vi "PECT - Scan_time gate_counter - PCI6071E.vi"() -> ()   [LabVIEW 2012]
uses:
  <vilib>/DAQmx/read.llb/DAQmx Read (Digital Bool 1Line 1Point).vi
  <vilib>/DAQmx/read.llb/DAQmx Read (Analog 2D DBL NChan NSamp).vi
  <vilib>/Instr/_visa.llb/VISA Configure Serial Port (Instr).vi
  <vilib>/DAQmx/create/channels.llb/DAQmx Create Channel (CO-Pulse Generation-Frequency).vi
  <vilib>/DAQmx/configure/timing.llb/DAQmx Timing (Implicit).vi
  <vilib>/DAQmx/configure/trigger.llb/DAQmx Start Trigger (Digital Edge).vi
  <vilib>/DAQmx/create/channels.llb/DAQmx Create Channel (DI-Digital Input).vi
  <vilib>/DAQmx/create/channels.llb/DAQmx Create Channel (AI-Voltage-Basic).vi
  <vilib>/DAQmx/configure/timing.llb/DAQmx Timing (Sample Clock).vi
  <vilib>/DAQmx/miscellaneous.llb/DAQmx Fill In Error Info.vi
  <resource>/objmgr/daqmx.rc
  <vilib>/Platform/NI_3dgraph.lvlib
  <vilib>/DAQmx/read.llb/DAQmx Read (Counter U32 1Chan 1Samp).vi
  <vilib>/DAQmx/create/channels.llb/DAQmx Create Channel (CI-Count Edges).vi
panel:
  in  "Counter Terminal":tag="/Dev3/PFI3"
  in  "Counter source":tag="Dev3/ctr1"
  in  "Tab Control 3":enum32{"Control", "Data Processing"}(tab)
  in  "Backdata online":bool caption="Scan"
  in  "Offset":bool
  in  "Open csv":bool
  in  "Scan":bool
  in  "Save Scan mode":bool caption="Save Process"
  in  "Gate 1":dbl=3.0
  in  "Gate 2":dbl=25.0
  in  "Stop Scan":bool
  in  "Right":bool
  in  "Left":bool
  in  "Front":bool
  in  "Back":bool
  in  "Home X":bool
  in  "Home Y":bool
  in  "Stop 3":bool
  in  "Emergency Stop":bool
  in  "Move Distance":dbl=5.0
  in  "Open tdms":bool
  in  "Pulse frequency":dbl=1000.0 format="%0.2p"
  in  "Pulser Cycles":i32=10
  in  "Sensor No.":i32
  in  "Graph":bool
  in  "Sensor Index":dbl[](array[numeric])=[5.0, 10.0, 12.0, 15.0, 19.0]
  in  "Inverse":bool caption="Scan"
  in  "Trim data":bool caption="Scan"
  in  "X-min":dbl
  in  "X-max":dbl
  in  "Y-min":dbl
  in  "Y-max":dbl
  in  "ViewMode":i32(ring) items=["cwViewXYPlane", "cwViewXZPlane", "cwViewYZPlane", "cwViewUserDefined"]
  in  "Plot style":i32(ring)=5 items=["cwLine"=1, "cwPoint"=2, "cwLinePoint"=3, "cwHiddenLine"=4, "cwSurface"=5, "cwSurfaceLine"=6, "cwSurfaceNormal"=7, "cwContourLine"=8, "cwSurfaceContour"=9]
  in  "Repair Line Col":bool
  in  "Repair Line Row":bool
  in  "Line Col":dbl=167.0
  in  "Line Row":dbl
  in  "low cutoff freq":dbl=40.0 format="%0.2f"
  in  "Filter":bool caption="Scan"
  in  "Backdata":bool caption="Scan"
  in  "Odd":bool caption="Scan"
  in  "DiffY":bool caption="Scan"
  in  "DiffX":bool caption="Scan"
  in  "ColorMapAutoScale":bool=TRUE
  in  "Max":dbl=0.6
  in  "Min":dbl=-0.8
  in  "Abs":bool caption="Scan"
  in  "Backindex":i32
  out "Completed":bool
  out "Start Pos. X":dbl=-55.0 format="%#.4f"
  out "Start. Pos.Y":dbl=-76.83 format="%#.4f"
  in  "Tab Control 2":T1(tab)
  out "Hall sensors signal":dbl[][](graph)
  out "Feature Extraction":dbl(graph)
  in  "3D Surface":refnum<k7>(container)
  out "Record path":path caption="selected path"
  out "Feature extraction scan":dbl[](graph)
  in  "Tab Control":T2(tab)=enum."          DAQ        "
  in  "Step X":dbl=0.5
  out "Move X":bool
  in  "Direction (+)":bool=TRUE
  in  "Step Y":dbl=1.0
  in  "Y-length":dbl=1.0
  in  "X-length":dbl=30.0
  in  "Save Speed":bool
  in  "Cur. Pos Y":dbl=18.8 format="%#.4f"
  in  "Cur. Pos X":dbl=-22.5 format="%#.4f"
  in  "Travel per Pulse (mm)":dbl=0.002
  in  "2 Rate":dbl=0.2
  in  "1 Rate":dbl=0.2
  in  "2 Min":dbl=1.0
  in  "1  Max":dbl=8.0
  in  "2 Max":dbl=8.0
  in  "1 Min":dbl=1.0
  in  "Parity":u16(ring) items=["None", "Odd", "Even", "Mark", "Space"]
  in  "stop bits":u16(ring)=10 items=["1.0"=10, "1.5"=15, "2.0"=20]
  in  "Data bits":u16=8 min=5 max=8 step=1
  in  "Baud Rate":u32=9600
  in  "COM Port":refnum<visa-resource-name>="COM3"
  out "No. X":i32
  out "No. Y":i32
  out "No. Data":i32
  out "Counter Status":bool
  out "Motor Pulse Count":i32
  in  "Digital Sampling Rate":dbl=1000.0
  in  "Digital Line":tag="Dev3/port0/line0"
  in  "AI Sample Clock":tag="/Dev3/Ctr0InternalOutput"
  in  "Pulse Counter":tag="Dev3/ctr0"
  in  "Edge":i32(ring)=10280 items=["Rising"=10280, "Falling"=10171]
  in  "Pulser edge terminal":tag="/Dev3/PFI0"
  out "Sample per Channel AI":dbl
  out "Actual Sample Rate":dbl=500000.0 format="%0.2f"
  in  "Physical Channel":tag="Dev3/ai0:31"
  in  "Min Voltage":dbl=-10.0
  in  "Max Voltage":dbl=10.0
  in  "Terminal Configuration":i32(ring)=10083 items=["default"=-1, "RSE"=10083, "NRSE"=10078, "Differential"=10106, "Pseudodifferential"=12529]
  in  "Sample Rate":dbl=30000.0
  in  "Save Scan mode 2":bool caption="Save Process"
  # "Pulse setting"
  # "Data Processing"
  # "Time gate = %T/2"
  # "Motor control"
  # "Color map"
  # "Process"
  # "Repair line"
  # "Hall Sensors Signal"
  # "Feature Extraction"
  # "COM  Setting"
  # "Speed  Setting"
  # "Scan  Setting"
  # "Pulser"
  # "Motor Trigger"
  # "Sensor  Channel"
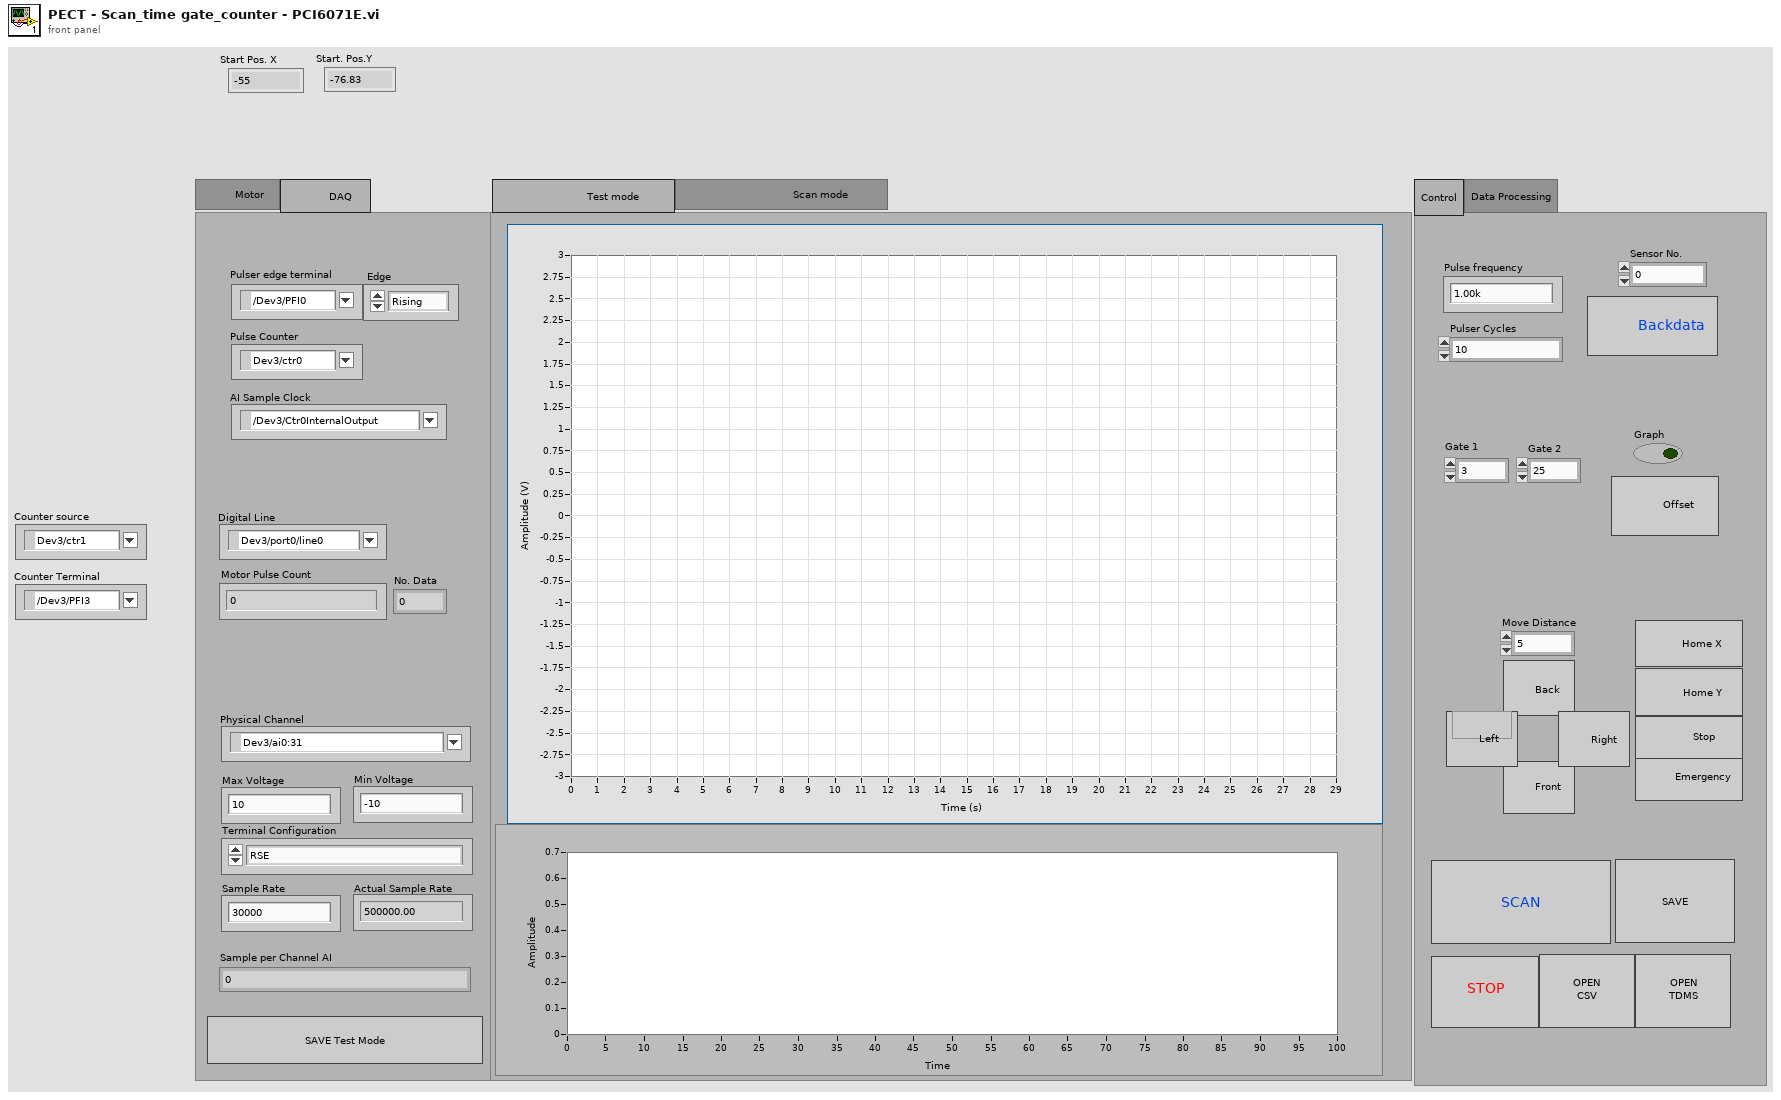
[diagram p1: front panel]
types:
  T1 = enum32{"                    Test mode                   ", "                          Scan mode                      "}
  T2 = enum32{"        Motor      ", "          DAQ        "}
  T3 = enum16{"No Scan", "Move X", "Wait to destination X", "Move Y", "Wait to destinatioin Y"}
  T4 = enum16{"open", "open or create", "create or replace", "create", "open (read-only)"}
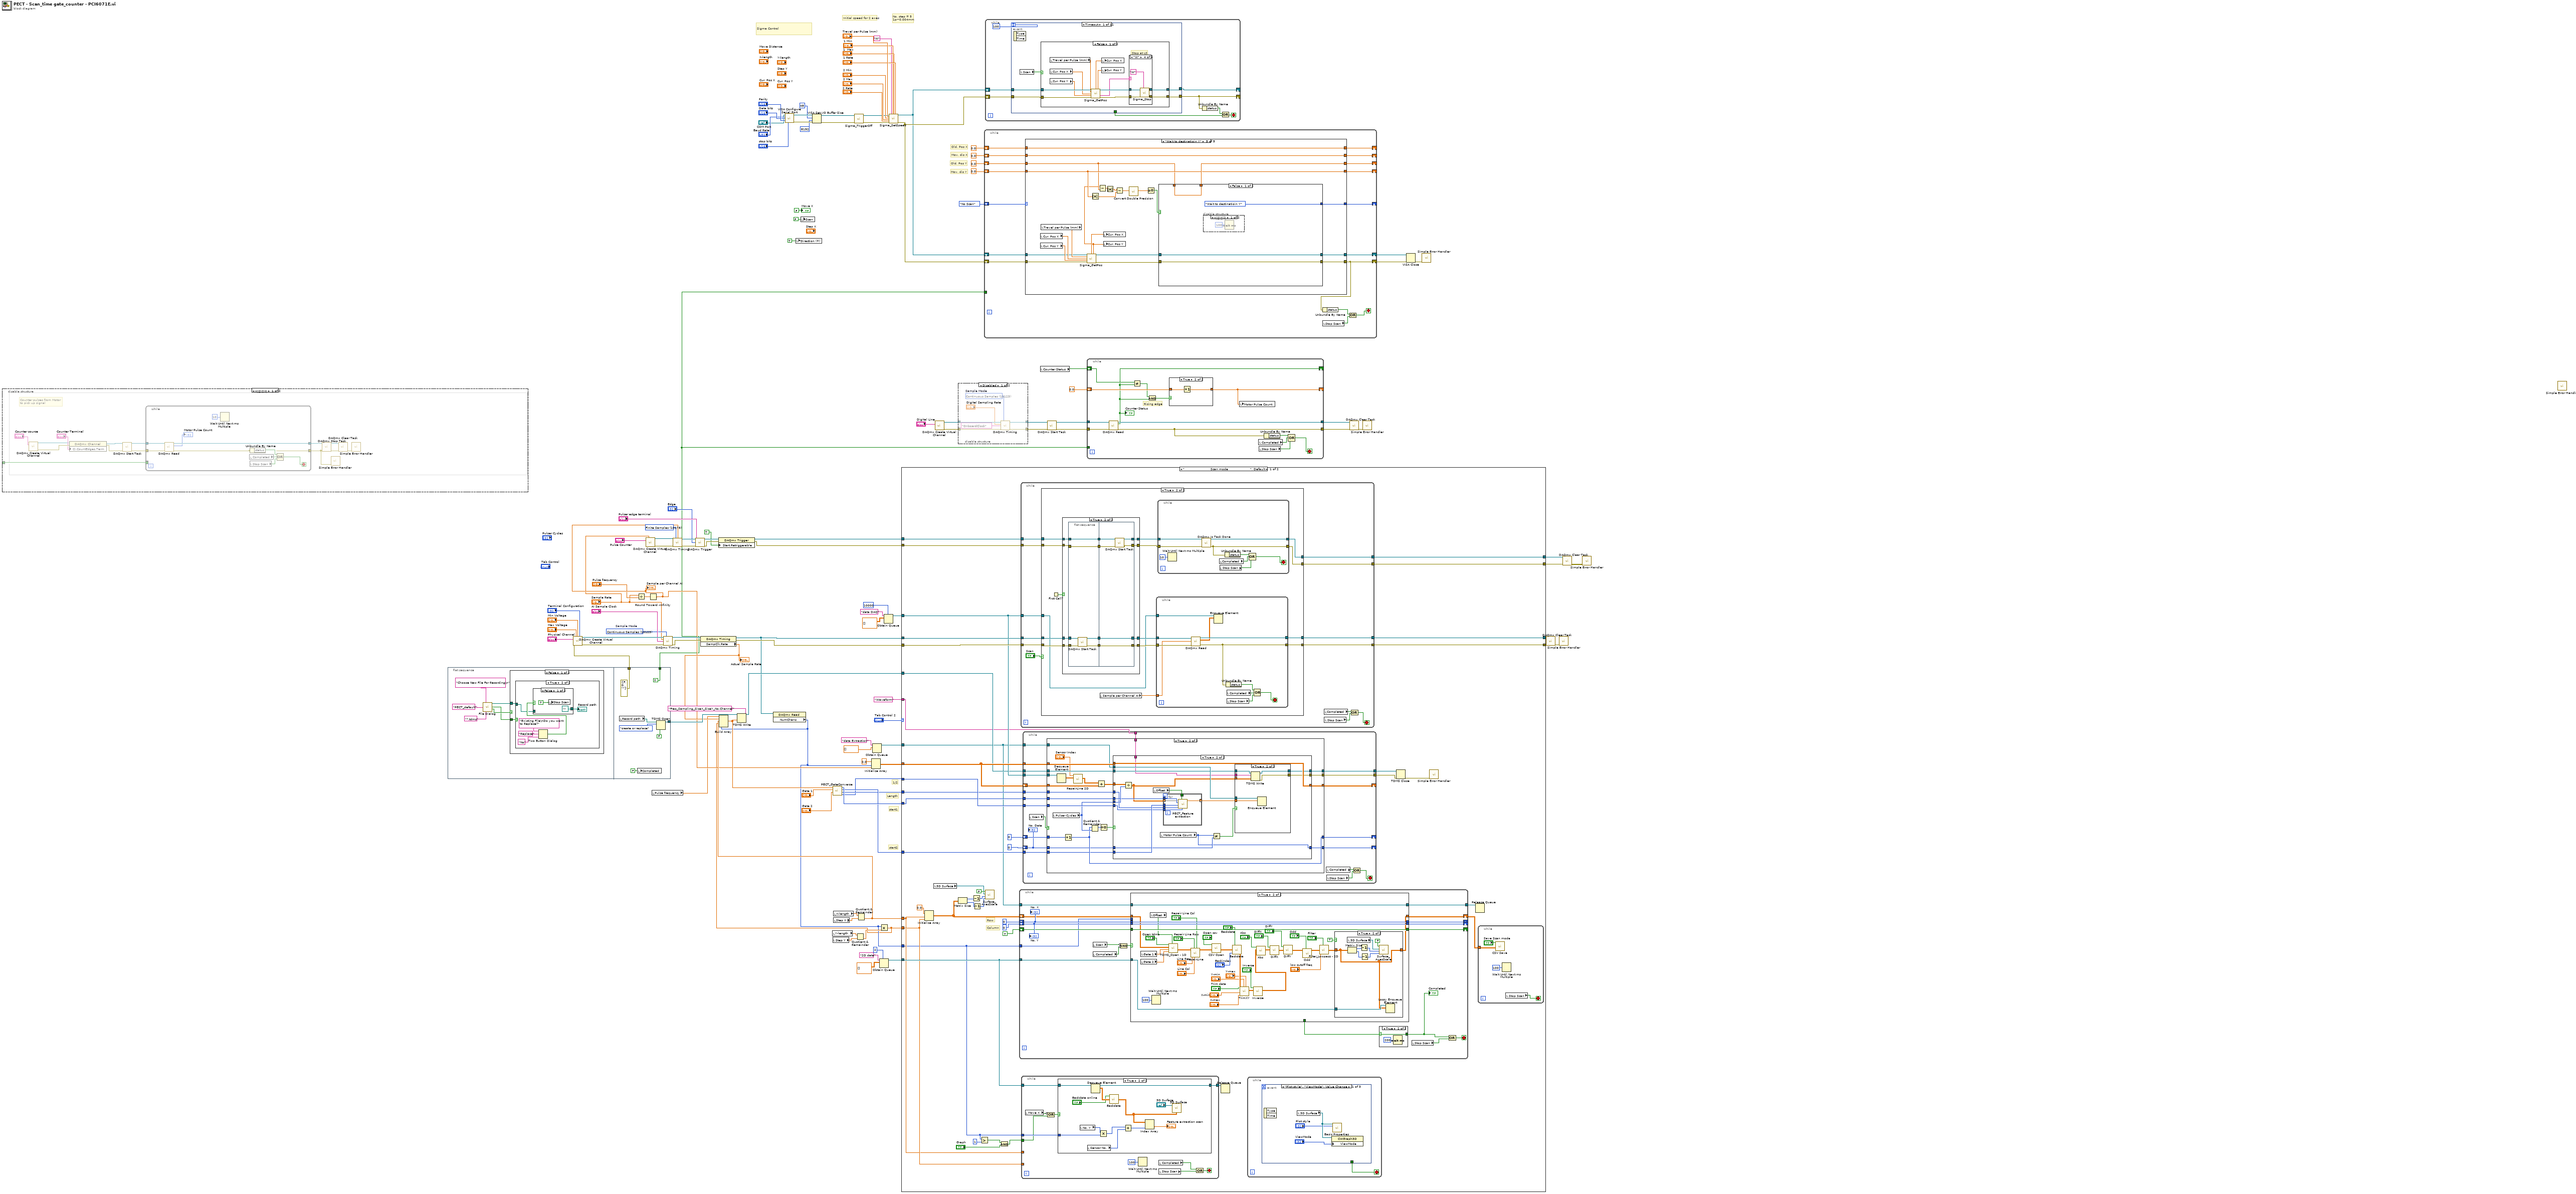
[diagram p0: block diagram]
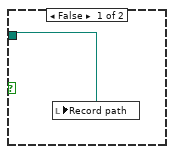
[diagram p5: hidden frame]
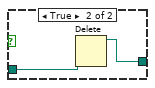
[diagram p6: hidden frame]
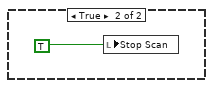
[diagram p7: hidden frame]
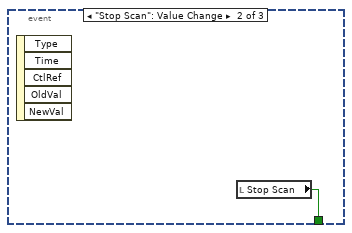
[diagram p8: hidden frame]
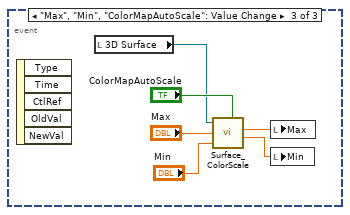
[diagram p9: hidden frame]
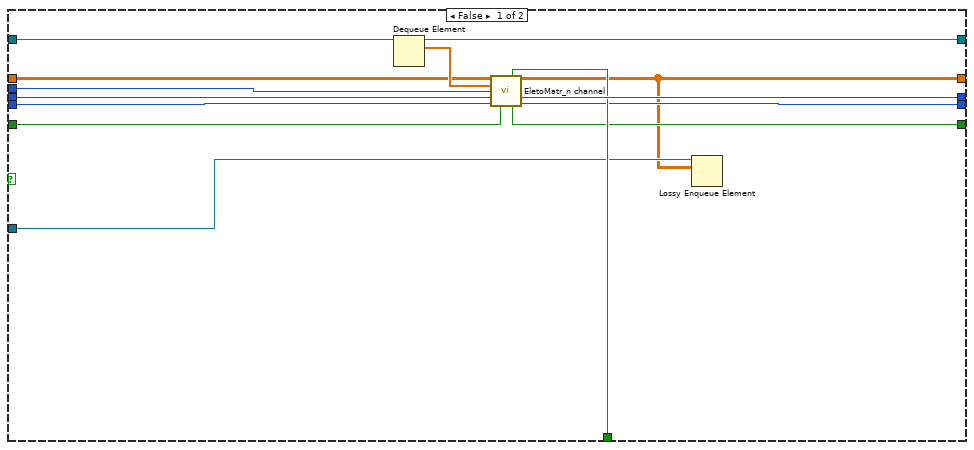
[diagram p12: hidden frame]
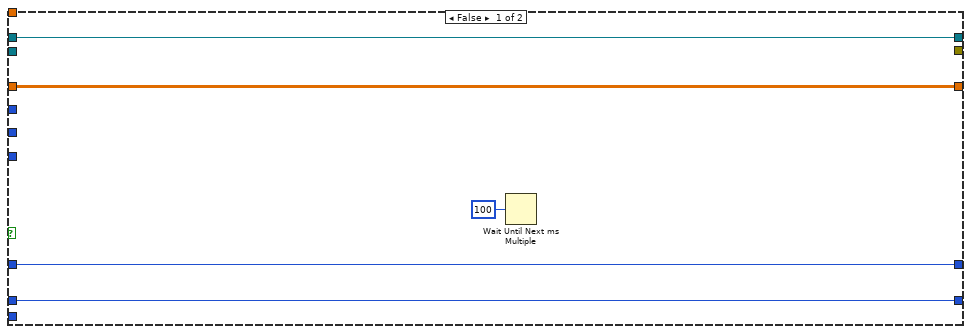
[diagram p16: hidden frame]
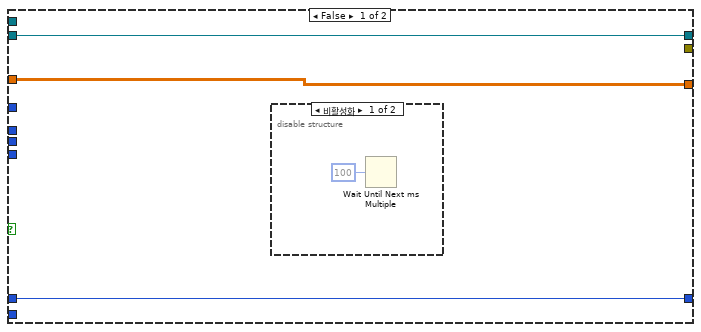
[diagram p17: hidden frame]
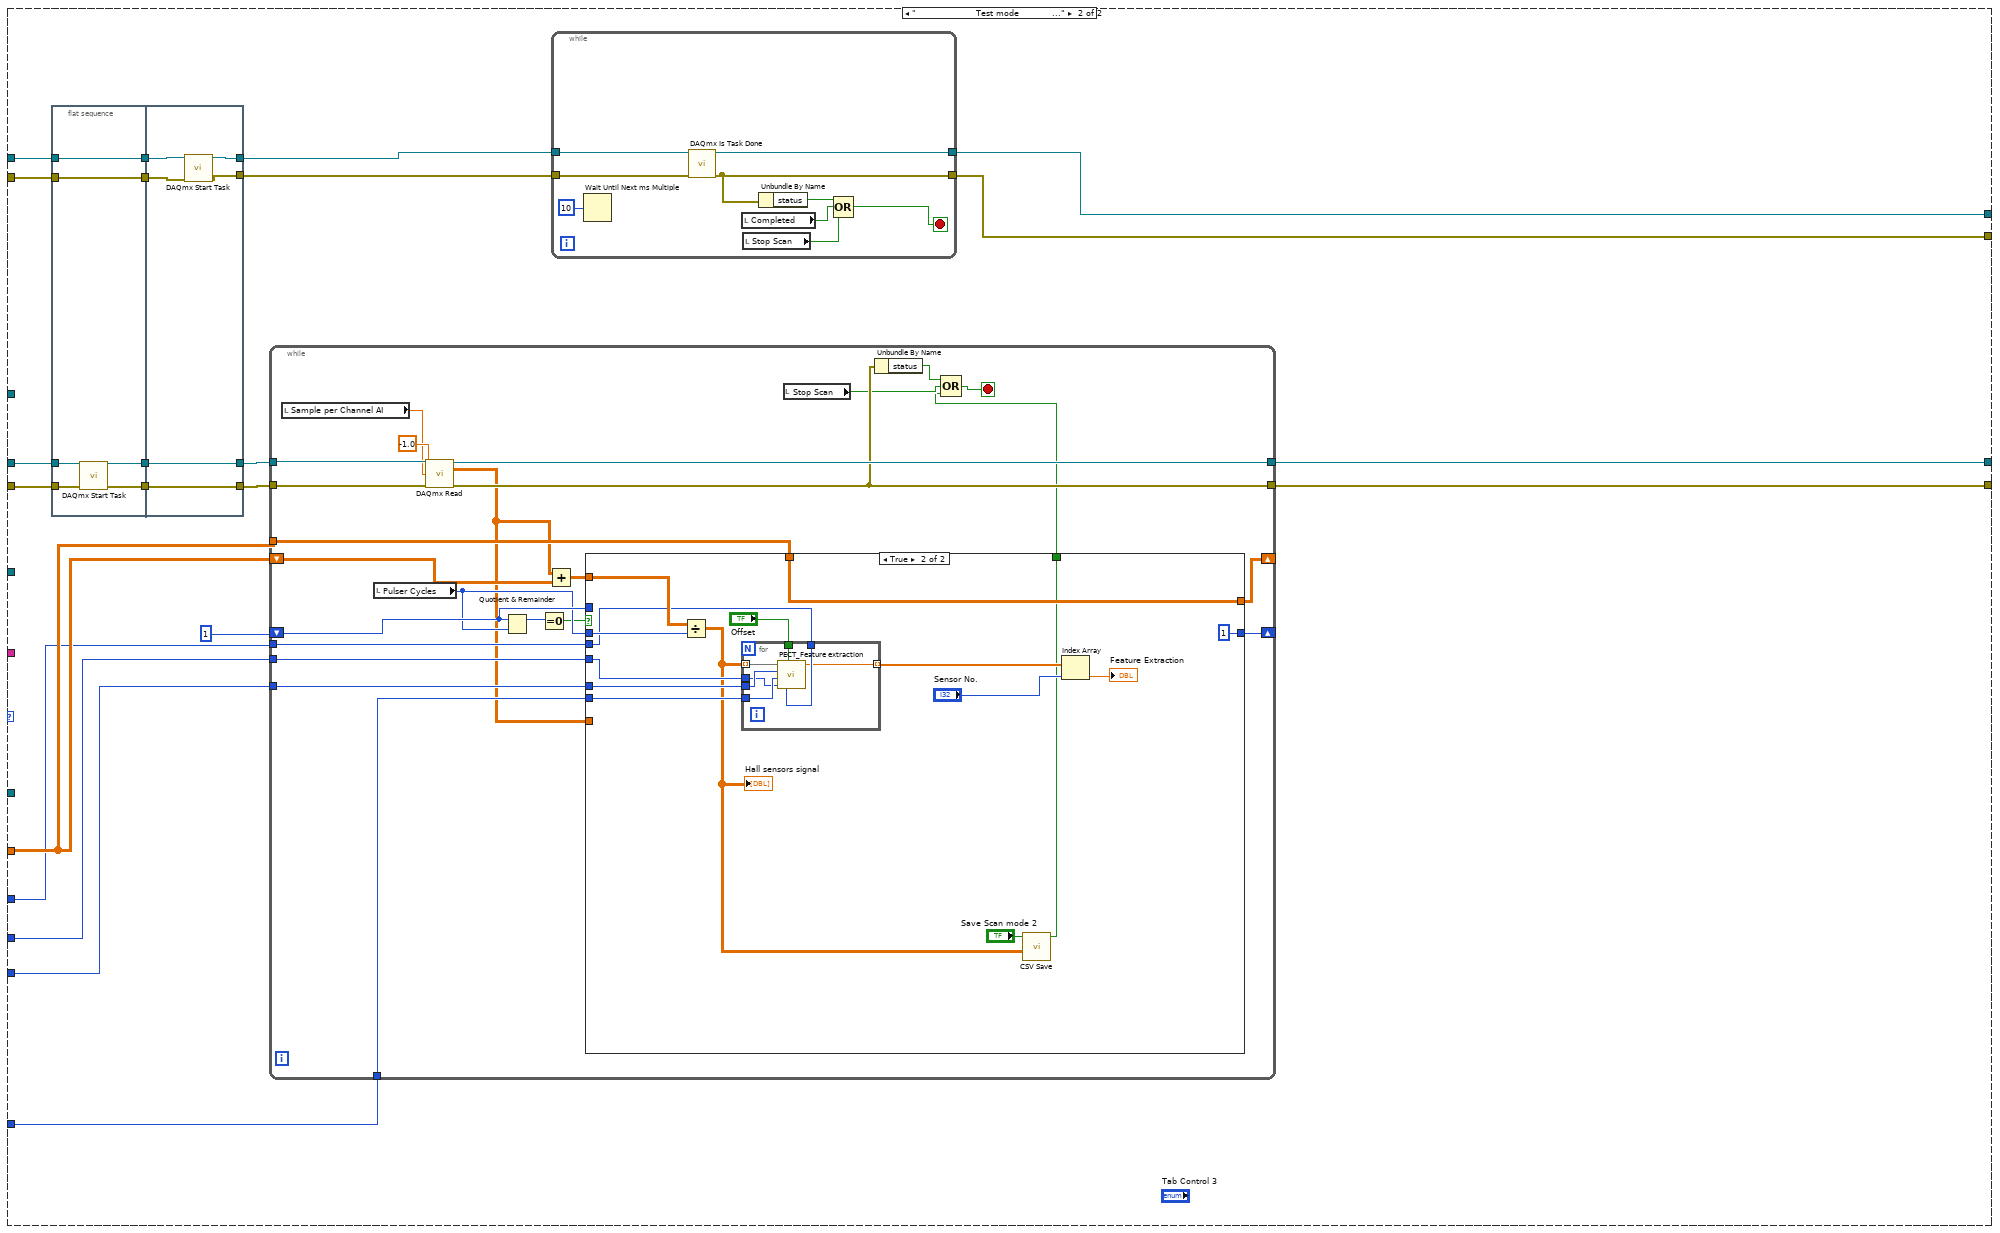
[diagram p20: hidden frame]
diagram:
  w38 = 10178 items=["Finite Samples"=10178, "Continuous Samples"=10123, "Hardware Timed Single Point"=12522] ("sample mode")
  w80 = 10123 items=["Finite Samples"=10178, "Continuous Samples"=10123, "Hardware Timed Single Point"=12522]  # Sample Mode
  # "1/2"
  # "start1"
  # "start2"
  # "Length"
  # "Mov. dis Y"
  # "Old. Pos Y"
  # "Mov. dis X"
  # "Old. Pos X"
  # "No. step = 5\n1p~0.004mm"
  # "Initial speed for 2 axes"
  # "Sigma Control"
  n1 = disable-structure shown="비활성화" {
    disable-tunnel: _ -> [w132 _]
    frame Disabled {
      # "Counter pulses from Motor\nto pick up signal"
      n2 = call-poly <vilib>:"DAQmx Create Virtual Channel.vi"("counter"="Counter source") -> ("task out"=w126:refnum<k21>, "error out"=w128:errorcluster)  [unwired: 13 in]
      n3 = property class="DAQmx Channel"(reference=w126, error in=w128, "CI.CountEdges.Term"="Counter Terminal") -> (reference out=w121:refnum<k21>, error out=w122:errorcluster)
      n4 = call <vilib>:"DAQmx Start Task.vi"("task/channels in"=w121, "error in"=w122) -> ("task out"=w123:refnum<k21>, "error out"=w120:errorcluster)  [unwired: 12 in]
      n5 = while {
        tunnel: w123 -> [w144]
        tunnel: w120 -> [w143]
        tunnel: [w136] -> w119
        tunnel: [w142] -> w129
        tunnel: [w135] -> _
        tunnel: w132 -> [w135]
        i -> [w133]
        stop <- w137 stop-if-true
        n6 = call-poly <vilib>:"DAQmx Read.vi"("task/channels in"=w144, "error in"=w143) -> ("task out"=w142:refnum<k21>, "data"=→"Motor Pulse Count":u32, "error out"=w136:errorcluster)  [unwired: 11 in]
        n7 = Wait Until Next ms Multiple(millisecond multiple=u32 10 ("milliseconds to wait")) -> ()  [unwired: 1 out]
        n8 = local read "Completed"() -> (w138:bool)
        n9 = Unbundle By Name(w136) -> ("status"=w140:bool)
        n10 = local read "Stop Scan"() -> (w139:bool)
        n11 = Compound Arithmetic op=OR(w140, w138, w139) -> (w137:bool)
      }
      n12 = call <vilib>:"DAQmx Stop Task.vi"("task/channels in"=w129, "error in"=w119) -> ("task out"=w131:refnum<k21>, "error out"=w130:errorcluster)  [unwired: 12 in]
      n13 = call <vilib>:"Simple Error Handler.vi"("error in (no error)"=w119) -> ()  [unwired: 4 in, 5 out]
      n14 = call <vilib>:"DAQmx Clear Task.vi"("task in"=w131, "error in"=w130) -> ("error out"=w124:errorcluster)  [unwired: 13 in]
      n15 = call <vilib>:"Simple Error Handler.vi"("error in (no error)"=w124) -> ()  [unwired: 4 in, 5 out]
    }
    frame Enabled {
    }
  }
  n16 = flat-sequence {
    tunnel: [w169] -> w65
    tunnel: [TRUE ("disable buffering (T)")] -> w4
    tunnel: [errorcluster {"status"=FALSE, "code"=0, "source"=""} ("error out")] -> w24
    frame #0 {
      n17 = call "File Dialog"("prompt"="Choose New File For Recording\n" ("button label"), "default name"="PECT_default", "pattern (all files)"="*.tdms") -> ("selected path"=w150:path, "exists"=w145:bool, "cancelled"=w146:bool)  [unwired: 9 in, 1 out]
      n18 = case shown="False" w146 {
        tunnel: w150 -> [w151 _]
        tunnel: w145 -> [w152 _]
        frame False {
          n19 = case shown="True" w152 {
            tunnel: w151 -> [w153 w154]
            frame False {
              n20 = local write "Record path"(w153) -> ()
            }
            frame True {
              n21 = Two Button Dialog(message="Existing File\nDo you want to Replace?", 1:"No" ("F button name (\"Cancel\")"), 2:"Replace" ("T button name (\"OK\")")) -> (T button?=w155:bool)
              n22 = case shown="False" w155 {
                tunnel: w154 -> [_ w163]
                tunnel: [path "" ("deleted path") w162] -> w156
                frame False {
                  n23 = local write "Stop Scan"(TRUE ("Exit")) -> ()
                }
                frame True {
                  n24 = Delete(path (use dialog)=w163) -> (deleted path=w162:path)  [unwired: 4 in, 2 out]
                }
              }
              "Record path" <- w156
            }
          }
        }
        frame True {
          n25 = local write "Stop Scan"(TRUE ("Exit")) -> ()
        }
      }
    }
    frame #1 {
      n26 = local read "Record path"() -> (w168:path)
      n27 = local write "Completed"(FALSE ("Completed")) -> ()
      n28 = TDMS Open(6:FALSE ("disable buffering (T)"), 10:T4."create or replace" ("operation"), 11:w168) -> (3:w169:refnum<k34>)  [unwired: 3 in, 1 out]
    }
  }
  n29 = call-poly <vilib>:"DAQmx Create Virtual Channel.vi"("maximum value"="Max Voltage", "minimum value"="Min Voltage", "input terminal configuration"="Terminal Configuration", "physical channels"="Physical Channel", "error in"=w24) -> ("task out"=w90:refnum<k21>, "error out"=w91:errorcluster)  [unwired: 9 in]
  n30 = Divide(x="Sample Rate", y="Pulse frequency") -> (x/y=w67:dbl)
  n31 = call-poly <vilib>:"DAQmx Create Virtual Channel.vi"("frequency"="Sample Rate", "counter"="Pulse Counter") -> ("task out"=w39:refnum<k21>, "error out"=w40:errorcluster)  [unwired: 7 in, 5 out]
  n32 = Round Toward -Infinity(1:w67) -> (0:w32:dbl)
  "Sample per Channel AI" <- w32
  n33 = local read "Pulse frequency"() -> (w27:dbl)
  n34 = call-poly <vilib>:"DAQmx Timing.vi"("task/channels in"=w90, "sample mode"=w80, "rate"="Sample Rate", "source"="AI Sample Clock", "error in"=w91) -> ("task out"=w41:refnum<k21>, "error out"=w92:errorcluster)  [unwired: 9 in]
  n35 = call-poly <vilib>:"DAQmx Timing.vi"("task/channels in"=w39, "sample mode"=w38, "samples per channel"=w32, "error in"=w40) -> ("task out"=w36:refnum<k21>, "error out"=w37:errorcluster)  [unwired: 10 out]
  n36 = call-poly <vilib>:"DAQmx Trigger.vi"("task/channels in"=w36, "source"="Pulser edge terminal", "edge"="Edge", "error in"=w37) -> ("task out"=w34:refnum<k21>, "error out"=w35:errorcluster)  [unwired: 10 out]
  n37 = property class="DAQmx Timing"(reference=w41, error in=w92) -> (reference out=w15:refnum<k21>, error out=w19:errorcluster, "SampClk.Rate"=w43:dbl)
  "Actual Sample Rate" <- w43
  n38 = property class="DAQmx Trigger"(reference=w34, error in=w35, "Start.Retriggerable"=TRUE) -> (reference out=w18:refnum<k21>, error out=w17:errorcluster)
  n39 = property class="DAQmx Read"(reference=w15) -> ("NumChans"=w23:u32)  [unwired: 1 in, 2 out]
  n40 = call-poly "VISA Configure Serial Port"("VISA resource name"="COM Port", "baud rate (9600)"="Baud Rate", "data bits (8)"="Data bits", "parity (0:none)"="Parity", "stop bits (10: 1 bit)"="stop bits") -> ("VISA resource name out"=w105:refnum<visa-resource-name>, "error out"=w111:errorcluster)  [unwired: 9 in]
  n41 = local write "Direction (+)"(TRUE ("Scan")) -> ()
  n42 = local write "Scan"(FALSE ("Scan")) -> ()
  n43 = VISA Set I/O Buffer Size(VISA resource name=w105, mask (16)=48, size (4096)=u32 8192, error in (no error)=w111) -> (VISA resource name out=w52:refnum<visa-resource-name>, error out=w51:errorcluster)
  n44 = local read "Y-length"() -> (w69:dbl)
  n45 = local read "Step Y"() -> (w70:dbl)
  n46 = local read "X-length"() -> (w72:dbl)
  n47 = local read "Step X"() -> (w71:dbl)
  n48 = call "Sigma_TriggerOff.vi"("error in (no error)"=w51, "VISA resource name"=w52) -> ("error out"=w49:errorcluster, "VISA resource name out"=w50:refnum<visa-resource-name>)  [unwired: 8 in]
  n49 = Quotient & Remainder(x=w69, y=w70) -> (floor(x/y)=w25:dbl)  [unwired: 1 out]
  n50 = Quotient & Remainder(x=w72, y=w71) -> (floor(x/y)=w63:dbl)  [unwired: 1 out]
  n51 = Initialize Array(0.0 ("element"), w23, w32) -> (w77:dbl[][])
  n52 = Obtain Queue(name (unnamed)="data Extraction", element data type=dbl[] [] ("data")) -> (queue out=w74:refnum<queue>)  [unwired: 3 in, 2 out]
  n53 = Obtain Queue(max queue size (-1, unlimited)=2 ("최대 큐 크기(-1,제한없음)"), name (unnamed)="2D data", element data type=dbl[][] [] ("initialized array")) -> (queue out=w45:refnum<queue>)  [unwired: 2 in, 2 out]
  n54 = Multiply(x=w23, y=w25) -> (x*y=w16:dbl)
  n55 = Build Array(w27, w43, w63, w16, w23) -> (w48:dbl[])
  n56 = TDMS Write(0:w65, 5:"Freq_Sampling_SizeX_SizeY_No.Channel" ("group name in (Untitled)"), 9:w48) -> (4:w64:refnum<k34>)  [unwired: 3 in, 3 out]
  n57 = call "PECT_GateConverse.vi"("Gate 2"="Gate 2", "Gate 1"="Gate 1", "Freq_Sampling_SizeX_SizeY"=w48) -> ("Length T/2"=w53:i32, "Length"=w54:i32, "Start 2"=w55:i32, "Start 1"=w56:i32)  [unwired: 5 in]
  n58 = Obtain Queue(max queue size (-1, unlimited)=10000, name (unnamed)="data DAQ", element data type=dbl[][] [] ("data")) -> (queue out=w76:refnum<queue>)  [unwired: 2 in, 2 out]
  n59 = call "Sigma_SetSpeed.vi"("VISA resource name"=w50, "Travel per Pulse (0.004mm)"="Travel per Pulse (mm)", "Min (1mm) 2"="2 Min", "Max (2mm) 2"="2 Max", "Rate (1mm) 2"="2 Rate", "error in (no error)"=w49, "Axis (1)"="W", "Min (1mm)"="1 Min", "Max (2mm)"="1  Max", "Rate (1mm)"="1 Rate") -> ("VISA resource name out"=w117:refnum<visa-resource-name>, "error out"=w118:errorcluster)  [unwired: 8 in]
  n60 = case shown="\"                          Scan mode                      \", Default" "Tab Control 2" {
    tunnel: w15 -> [w215 w518]
    tunnel: [w214 w530] -> w83
    tunnel: [w213 w529] -> w82
    tunnel: w77 -> [w210 w528]
    tunnel: w19 -> [w212 w517]
    tunnel: w53 -> [w211 w527]
    tunnel: w76 -> [w209 _]
    tunnel: w74 -> [w189 _]
    tunnel: w63 -> [w184 _]
    tunnel: w16 -> [w185 _]
    tunnel: w54 -> [w197 w525]
    tunnel: w56 -> [w196 w524]
    tunnel: w55 -> [w195 w523]
    tunnel: w64 -> [w194 _]
    tunnel: "Waveform" ("group name in (Untitled)") -> [w191 _]
    tunnel: w45 -> [w186 _]
    tunnel: w23 -> [w176 _]
    tunnel: [w181 w510] -> w21
    tunnel: [w180 w509] -> w20
    tunnel: w18 -> [w179 w514]
    tunnel: w17 -> [w178 w513]
    frame "                          Scan mode                      ", Default {
      # "Column"
      # "Row"
      n61 = Initialize Array(0.0 ("element"), w184, w185) -> (w177:dbl[][])
      n62 = local read "3D Surface"() -> (w198:refnum<k7>)
      n63 = Matrix Size(0:w177) -> (1:w203:i32, 2:w204:i32)
      n64 = Decrement(x=w203) -> (x-1=w207:i32)
      n65 = Decrement(x=w204) -> (x-1=w206:i32)
      n66 = Greater?(x=w176, y=u32 1) -> (0:w174:bool)
      n67 = call "Surface_AxesScale.vi"("Y-axis Max"=w206, "X-axis max"=w207, "3D Surface"=w198, "Auto Scale"=FALSE) -> ()  [unwired: 8 in]
      n68 = Compound Arithmetic op=AND(w174, "Graph") -> (w172:bool)
      n69 = while {
        shift-right: [w270] -> _
        shift-left: 0 -> [w272]
        shift-right: [w269] -> _
        shift-left: 0 -> [w271]
        tunnel: w189 -> [w268]
        shift-right: [w260] -> w182
        shift-left: w177 -> [w267]
        shift-right: [w263] -> _
        shift-left: TRUE ("Output Direction") -> [w264]
        tunnel: w186 -> [w262]
        tunnel: [w261] -> w187
        tunnel: w176 -> [w256]
        stop <- w265 stop-if-true
        n70 = local read "Scan"() -> (w259:bool)
        n71 = local read "Completed"() -> (w258:bool)
        n72 = Compound Arithmetic op=AND(invert w259, invert w258) -> (w257:bool)
        n73 = case shown="True" w257 {
          tunnel: w272 -> [w289 w332]
          tunnel: w271 -> [w288 w331]
          tunnel: [w287 w332] -> w270
          tunnel: [w282 w331] -> w269
          tunnel: w268 -> [w286 w323]
          tunnel: w267 -> [w277 w328]
          tunnel: [w280 w310] -> w260
          tunnel: [w285 _] -> w255
          tunnel: w264 -> [w284 w330]
          tunnel: [w283 w330] -> w263
          tunnel: w262 -> [w281 w312]
          tunnel: [w276 w323] -> w261
          tunnel: w256 -> [w278 _]
          frame False {
            n74 = Dequeue Element(queue=w286) -> (queue out=w276:refnum<queue>, element=w279:dbl[])  [unwired: 2 in, 2 out]
            n75 = call "EletoMatr_n channel.vi"("Input Array X"=w277, "Input data"=w279, "No. channels"=w278, "In Row"=w289, "In Column"=w288, "Input Direction"=w284) -> ("Completed"=w285:bool, "Out Array X"=w280:dbl[][], "Out Row"=w287:i32, "Output Direction"=w283:bool, "Out Column"=w282:i32)  [unwired: 5 in]
            n76 = Lossy Enqueue Element(queue=w281, element=w280) -> ()  [unwired: 1 in, 4 out]
          }
          frame True {
            n77 = local read "Gate 1"() -> (w327:dbl)
            n78 = local read "Gate 2"() -> (w326:dbl)
            n79 = local read "Offset"() -> (w317:bool)
            n80 = Wait Until Next ms Multiple(millisecond multiple=u32 100 ("ms 배수")) -> ()  [unwired: 1 out]
            n81 = call "TDMS_Open - 1D.vi"("Offset"=w317, "Gate 2"=w326, "Gate 1"=w327, "Input 2D"=w328, "Open"="Open tdms") -> ("Output 2D"=w304:dbl[][])  [unwired: 5 in, 1 out]
            n82 = call "RepairLine.vi"("Repair Line Col"="Repair Line Col", "Repair Line Row"="Repair Line Row", "Line Col"="Line Col", "Line Row"="Line Row", "Array In"=w304) -> ("Array Repaired"=w303:dbl[][])  [unwired: 6 in]
            n83 = call "CSV Open.vi"("2D Array In"=w303, "Open"="Open csv") -> ("2D Array Out"=w311:dbl[][])  [unwired: 9 in]
            n84 = call "Backdata.vi"("Backindex"="Backindex", "Array in"=w311, "Backdata"="Backdata") -> ("Array out"=w298:dbl[][])
            n85 = call "TrimXY.vi"("X-max"="Y-max", "X-min"="Y-min", "Y-max"="X-max", "Y-min"="X-min", "Array In"=w298, "Trim data"="Trim data") -> ("Array Trim Out"=w292:dbl[][])  [unwired: 5 in]
            n86 = call "Inverse.vi"(10:"Inverse"=w292, 11:"Inverse"="Inverse") -> ("Array out"=w290:dbl[][])  [unwired: 9 in]
            n87 = call "Abs.vi"("Input"=w290, "Abs"="Abs") -> ("Array out"=w316:dbl[][])  [unwired: 9 in]
            n88 = call "DiffX.vi"("Array in"=w316, "DiffX"="DiffX") -> ("Array out"=w321:dbl[][])  [unwired: 1 in]
            n89 = call "DiffY.vi"("Array in"=w321, "DiffY"="DiffY") -> ("Array out"=w319:dbl[][])  [unwired: 1 in]
            n90 = call "Odd.vi"("Odd"="Odd", "Array In"=w319) -> ("Array Out"=w308:dbl[][])  [unwired: 9 in]
            n91 = call "Filter_Lowpass - 2D.vi"("Filter"="Filter", "Input 2D"=w308, "low cutoff freq: fl"="low cutoff freq") -> ("Output"=w307:dbl[][])  [unwired: 6 in]
            n92 = case shown="True" TRUE {
              tunnel: w307 -> [w333 w334]
              tunnel: [w333 w334] -> w310
              tunnel: w312 -> [_ w335]
              frame False {
              }
              frame True {
                n93 = local read "3D Surface"() -> (w339:refnum<k7>)
                n94 = Matrix Size(0:w334) -> (1:w340:i32, 2:w337:i32)
                n95 = Decrement(x=w340) -> (x-1=w338:i32)
                n96 = Decrement(x=w337) -> (x-1=w336:i32)
                n97 = call "Surface_AxesScale.vi"("Y-axis Max"=w336, "X-axis max"=w338, "3D Surface"=w339, "Auto Scale"=FALSE) -> ()  [unwired: 8 in]
                n98 = Lossy Enqueue Element(queue=w335, element=w334) -> ()  [unwired: 1 in, 4 out]
              }
            }
          }
        }
        n99 = case shown="True" w255 {
          selector: w255 -> [w273 w274]
          tunnel: [w273 w274] -> w254
          frame False {
          }
          frame True {
            n100 = Wait (ms)(milliseconds to wait=u32 200) -> ()  [unwired: 1 out]
          }
        }
        "Completed" <- w254
        n101 = local read "Stop Scan"() -> (w266:bool)
        n102 = Compound Arithmetic op=OR(w254, w266) -> (w265:bool)
        "No. Y" <- w271
        "No. X" <- w272
      }
      n103 = while {
        tunnel: w215 -> [w354]
        tunnel: [w353] -> w214
        tunnel: [w352] -> w213
        tunnel: w212 -> [w351]
        tunnel: w209 -> [w350]
        tunnel: [w345] -> w181
        tunnel: [w344] -> w180
        tunnel: w179 -> [w343]
        tunnel: w178 -> [w342]
        stop <- w346 stop-if-true
        n104 = case shown="True" "Scan" {
          tunnel: w354 -> [w358 w369]
          tunnel: [w358 w373] -> w353
          tunnel: [w357 w372] -> w352
          tunnel: w351 -> [w357 w368]
          tunnel: w350 -> [_ w361]
          tunnel: [w356 w371] -> w345
          tunnel: [w355 w370] -> w344
          tunnel: w343 -> [w356 w365]
          tunnel: w342 -> [w355 w364]
          frame False {
          }
          frame True {
            n105 = First Call?() -> (First Call?: T/F=w360:bool)
            n106 = case shown="True" w360 {
              tunnel: w369 -> [w375 w385]
              tunnel: w368 -> [w374 w384]
              tunnel: [w375 w383] -> w367
              tunnel: [w374 w382] -> w366
              tunnel: w365 -> [w377 w381]
              tunnel: w364 -> [w376 w380]
              tunnel: [w377 w379] -> w363
              tunnel: [w376 w378] -> w362
              frame False {
              }
              frame True {
                n107 = flat-sequence {
                  tunnel: w385 -> [w395]
                  tunnel: w384 -> [w394]
                  tunnel: [w393] -> w389
                  tunnel: [w392] -> w388
                  tunnel: [w391] -> w387
                  tunnel: w381 -> [w391]
                  tunnel: w380 -> [w390]
                  tunnel: [w390] -> w386
                  tunnel: [w400] -> w382
                  tunnel: [w401] -> w383
                  tunnel: w389 -> [w401]
                  tunnel: w388 -> [w400]
                  tunnel: w387 -> [w399]
                  tunnel: w386 -> [w398]
                  tunnel: [w397] -> w379
                  tunnel: [w396] -> w378
                  frame #0 {
                    n108 = call <vilib>:"DAQmx Start Task.vi"("task/channels in"=w395, "error in"=w394) -> ("task out"=w393:refnum<k21>, "error out"=w392:errorcluster)  [unwired: 12 in]
                  }
                  frame #1 {
                    n109 = call <vilib>:"DAQmx Start Task.vi"("task/channels in"=w399, "error in"=w398) -> ("task out"=w397:refnum<k21>, "error out"=w396:errorcluster)  [unwired: 12 in]
                  }
                }
              }
            }
            n110 = local read "Sample per Channel AI"() -> (w359:dbl)
            n111 = while {
              tunnel: [w421] -> w373
              tunnel: [w420] -> w372
              tunnel: w361 -> [w419]
              tunnel: w367 -> [w414]
              tunnel: w366 -> [w413]
              tunnel: w359 -> [w411]
              stop <- w415 stop-if-true
              n112 = call-poly <vilib>:"DAQmx Read.vi"("task/channels in"=w414, "number of samples per channel"=w411, "error in"=w413) -> ("task out"=w421:refnum<k21>, "data"=w412:dbl[][], "error out"=w420:errorcluster)  [unwired: 10 in]
              n113 = Enqueue Element(queue=w419, element=w412) -> ()  [unwired: 2 in, 3 out]
              n114 = Unbundle By Name(w420) -> ("status"=w416:bool)
              n115 = local read "Completed"() -> (w418:bool)
              n116 = local read "Stop Scan"() -> (w417:bool)
              n117 = Compound Arithmetic op=OR(w416, w418, w417) -> (w415:bool)
            }
            n118 = while {
              tunnel: w363 -> [w410]
              tunnel: w362 -> [w409]
              tunnel: [w407] -> w370
              tunnel: [w406] -> w371
              stop <- w404 stop-if-true
              n119 = Wait Until Next ms Multiple(millisecond multiple=u32 10) -> ()  [unwired: 1 out]
              n120 = call <vilib>:"DAQmx Is Task Done.vi"("task/channels in"=w410, "error in"=w409) -> ("task out"=w406:refnum<k21>, "error out"=w407:errorcluster)  [unwired: 12 out]
              n121 = local read "Completed"() -> (w403:bool)
              n122 = local read "Stop Scan"() -> (w402:bool)
              n123 = Unbundle By Name(w407) -> ("status"=w405:bool)
              n124 = Compound Arithmetic op=OR(w405, w403, w402) -> (w404:bool)
            }
          }
        }
        n125 = local read "Completed"() -> (w347:bool)
        n126 = local read "Stop Scan"() -> (w348:bool)
        n127 = Compound Arithmetic op=OR(w347, w348) -> (w346:bool)
      }
      n128 = while {
        tunnel: w186 -> [w234]
        tunnel: w185 -> [_]
        tunnel: w184 -> [_]
        tunnel: [w237] -> w183
        tunnel: w176 -> [w236]
        tunnel: w172 -> [w232]
        stop <- w238 stop-if-true
        n129 = local read "Move X"() -> (w233:bool)
        n130 = Compound Arithmetic op=OR(invert w233, w232) -> (w231:bool)
        n131 = case shown="True" w231 {
          tunnel: [w241 w251] -> w237
          tunnel: w236 -> [_ w249]
          tunnel: w234 -> [w241 w245]
          frame False {
          }
          frame True {
            n132 = local read "No. Y"() -> (w250:i32)
            n133 = local read "Sensor No."() -> (w247:i32)
            n134 = Dequeue Element(queue=w245) -> (queue out=w251:refnum<queue>, element=w244:dbl[][])  [unwired: 2 in, 2 out]
            n135 = Multiply(x=w250, y=w249) -> (x*y=w248:u32)
            n136 = call "Backdata.vi"("Array in"=w244, "Backdata"="Backdata online") -> ("Array out"=w243:dbl[][])  [unwired: 1 in]
            n137 = Add(x=w248, y=w247) -> (x+y=w246:u32)
            n138 = Index Array(array=w243, index (col)=w246) -> (element=→"Feature extraction scan":dbl[])  [unwired: 1 in]
            n139 = call <vilib>:"3D Surface.vi"("z matrix"=w243, "3D graph"="3D Surface") -> ()  [unwired: 8 in, 2 out]
          }
        }
        n140 = Wait Until Next ms Multiple(millisecond multiple=u32 100 ("ms 배수")) -> ()  [unwired: 1 out]
        n141 = local read "Completed"() -> (w235:bool)
        n142 = local read "Stop Scan"() -> (w239:bool)
        n143 = Compound Arithmetic op=OR(w235, w239) -> (w238:bool)
      }
      n144 = while {
        shift-right: [w438] -> _
        shift-left: w210 -> [w442]
        tunnel: w210 -> [w441]
        tunnel: w211 -> [w440]
        tunnel: w209 -> [w439]
        tunnel: w189 -> [w437]
        shift-right: [w434] -> _
        shift-left: 0 -> [w435]
        tunnel: w197 -> [w433]
        tunnel: w196 -> [w432]
        tunnel: w195 -> [w431]
        tunnel: w194 -> [w430]
        tunnel: [w429] -> w193
        tunnel: [w428] -> w192
        tunnel: w191 -> [w427]
        shift-right: [w426] -> _
        shift-left: 0 -> [w422]
        stop <- w423 stop-if-true
        n145 = local read "Scan"() -> (w436:bool)
        n146 = case shown="True" w436 {
          tunnel: w442 -> [w447 w463]
          tunnel: w441 -> [_ w468]
          tunnel: w440 -> [_ w467]
          tunnel: w439 -> [_ w466]
          tunnel: [w447 w465] -> w438
          tunnel: w437 -> [_ w464]
          tunnel: w435 -> [w446 w461]
          tunnel: [w446 w460] -> w434
          tunnel: w433 -> [_ w459]
          tunnel: w432 -> [_ w458]
          tunnel: w431 -> [_ w457]
          tunnel: w430 -> [w444 w456]
          tunnel: [w444 w455] -> w429
          tunnel: [_ w454] -> w428
          tunnel: w427 -> [_ w453]
          tunnel: w422 -> [w443 w452]
          tunnel: [w443 w451] -> w426
          frame False {
            n147 = Wait Until Next ms Multiple(millisecond multiple=u32 100 ("ms 배수")) -> ()  [unwired: 1 out]
          }
          frame True {
            n148 = local read "Pulser Cycles"() -> (w462:i32)
            n149 = Dequeue Element(queue=w466) -> (element=w450:dbl[][])  [unwired: 2 in, 3 out]
            n150 = Increment(x=w461) -> (x+1=w460:i32)
            n151 = call "RepairLine 2D.vi"("Array in"=w450, "Sensor Index"="Sensor Index") -> ("Array Out"=w448:dbl[][])  [unwired: 9 in]
            n152 = Quotient & Remainder(x=w460, y=w462) -> (x-y*floor(x/y)=w469:i32)  [unwired: 1 out]
            n153 = Add(x=w448, y=w463) -> (x+y=w471:dbl[][])
            n154 = Equal To 0?(x=w469) -> (x = 0?=w470:bool)
            n155 = case shown="True" w470 {
              tunnel: w462 -> [_ w492]
              tunnel: w471 -> [w474 w490]
              tunnel: [w474 w493] -> w465
              tunnel: w468 -> [_ w493]
              tunnel: w467 -> [_ w486]
              tunnel: w464 -> [_ w491]
              tunnel: w459 -> [_ w487]
              tunnel: w458 -> [_ w489]
              tunnel: w457 -> [_ w488]
              tunnel: w456 -> [w473 w482]
              tunnel: [w473 w479] -> w455
              tunnel: [_ w478] -> w454
              tunnel: w453 -> [_ w481]
              tunnel: w452 -> [w472 w483]
              tunnel: [w472 w477] -> w451
              frame False {
                n156 = disable-structure shown="비활성화" {
                  frame Disabled {
                    n157 = Wait Until Next ms Multiple(millisecond multiple=u32 100 ("ms 배수")) -> ()  [unwired: 1 out]
                  }
                  frame Enabled {
                  }
                }
              }
              frame True {
                n158 = Divide(x=w490, y=w492) -> (x/y=w480:dbl[][])
                n159 = local read "Offset"() -> (w485:bool)
                n160 = local read "Motor Pulse Count"() -> (w477:i32)
                n161 = for {
                  tunnel: w489 -> [w500]
                  tunnel: w488 -> [w499]
                  tunnel: w487 -> [w498]
                  tunnel: w486 -> [w497]
                  tunnel: w485 -> [w496]
                  tunnel: [w495] -> w484 mode=indexing
                  tunnel: w480 -> [w494] mode=indexing
                  n162 = call "PECT_Feature extraction.vi"("Length T/2"=w497, "Offset"=w496, "Length"=w498, "Start 2"=w499, "Start 1"=w500, "Pulse signal in"=w494) -> ("Feature extraction out"=w495:dbl)  [unwired: 5 in]
                }
                n163 = Not Equal?(x=w477, y=w483) -> (x != y?=w476:bool)
                n164 = case shown="True" w476 {
                  tunnel: w491 -> [_ w508]
                  tunnel: w484 -> [_ w507]
                  tunnel: w482 -> [w501 w506]
                  tunnel: w481 -> [_ w505]
                  tunnel: w480 -> [_ w504]
                  tunnel: [w501 w503] -> w479
                  tunnel: [_ w502] -> w478
                  frame False {
                  }
                  frame True {
                    n165 = TDMS Write(0:w506, 5:w505, 9:w504) -> (4:w503:refnum<k34>, 15:w502:errorcluster)  [unwired: 3 in, 2 out]
                    n166 = Enqueue Element(queue=w508, element=w507) -> ()  [unwired: 2 in, 3 out]
                  }
                }
              }
            }
          }
        }
        n167 = local read "Completed"() -> (w425:bool)
        n168 = local read "Stop Scan"() -> (w424:bool)
        n169 = Compound Arithmetic op=OR(w425, w424) -> (w423:bool)
        "No. Data" <- w422
      }
      n170 = Release Queue(queue=w183) -> ()  [unwired: 2 in, 3 out]
      n171 = while {
        stop <- w220 stop-if-true
        n172 = event shown="[0] \"Plot style\", \"ViewMode\": Value Change" {
          selector: _ -> [_ _ _]
          dyn-events: _ -> [_ _ _]
          timeout: _ -> [_ _ _]
          tunnel: [_ w224 _] -> w220
          event "Plot style", "ViewMode": Value Change {
            n173 = event-data() -> ()  [unwired: 1 in, 2 out]
            n174 = local read "3D Surface"() -> (w223:refnum<k7>)
            n175 = property class="CWGraph3D"(reference=w223, "ViewMode"="ViewMode") -> ()  [unwired: 1 in, 2 out]
            n176 = call <vilib>:"Basic Properties.vi"("3D graph"=w223, "plot style"="Plot style") -> ()  [unwired: 12 in, 2 out]
          }
          event "Stop Scan": Value Change {
            n177 = event-data() -> ()  [unwired: 1 in, 5 out]
            n178 = local read "Stop Scan"() -> (w224:bool)
          }
          event "Max", "Min", "ColorMapAutoScale": Value Change {
            n179 = event-data() -> ()  [unwired: 1 in, 5 out]
            n180 = local read "3D Surface"() -> (w225:refnum<k7>)
            n181 = call "Surface_ColorScale.vi"("ColorMapAutoScale"="ColorMapAutoScale", "Min"="Min", "Max"="Max", "3D Surface_"=w225) -> ("Min 2"=w229:dbl, "Max 2"=w228:dbl)  [unwired: 1 in, 2 out]
            n182 = local write "Max"(w228) -> ()
            n183 = local write "Min"(w229) -> ()
          }
        }
      }
      n184 = TDMS Close(8:w192, 11:w193) -> (0:w190:errorcluster)  [unwired: 1 out]
      n185 = call <vilib>:"Simple Error Handler.vi"("error in (no error)"=w190) -> ()  [unwired: 2 in, 7 out]
      n186 = Release Queue(queue=w187) -> ()  [unwired: 2 in, 3 out]
      n187 = while {
        tunnel: w182 -> [w218]
        stop <- w217 stop-if-true
        n188 = call "CSV Save.vi"("Array"=w218, "Save Button"="Save Scan mode") -> ()  [unwired: 9 in, 1 out]
        n189 = Wait Until Next ms Multiple(millisecond multiple=u32 100 ("ms 배수")) -> ()  [unwired: 1 out]
        n190 = local read "Stop Scan"() -> (w217:bool)
      }
    }
    frame "                    Test mode                   " {
      n191 = flat-sequence {
        tunnel: w518 -> [w536]
        tunnel: w517 -> [w535]
        tunnel: [w534] -> w522
        tunnel: [w533] -> w521
        tunnel: [w532] -> w520
        tunnel: w514 -> [w532]
        tunnel: w513 -> [w531]
        tunnel: [w531] -> w519
        tunnel: [w541] -> w515
        tunnel: [w542] -> w516
        tunnel: w522 -> [w542]
        tunnel: w521 -> [w541]
        tunnel: w520 -> [w540]
        tunnel: w519 -> [w539]
        tunnel: [w538] -> w512
        tunnel: [w537] -> w511
        frame #0 {
          n192 = call <vilib>:"DAQmx Start Task.vi"("task/channels in"=w536, "error in"=w535) -> ("task out"=w534:refnum<k21>, "error out"=w533:errorcluster)  [unwired: 12 in]
        }
        frame #1 {
          n193 = call <vilib>:"DAQmx Start Task.vi"("task/channels in"=w540, "error in"=w539) -> ("task out"=w538:refnum<k21>, "error out"=w537:errorcluster)  [unwired: 12 in]
        }
      }
      n194 = while {
        tunnel: w516 -> [w559]
        tunnel: w515 -> [w558]
        tunnel: [w574] -> w529
        tunnel: [w575] -> w530
        shift-right: [w571] -> _
        shift-left: w528 -> [w572]
        tunnel: w528 -> [w570]
        tunnel: w527 -> [w568]
        shift-right: [w566] -> _
        shift-left: 1 ("Average") -> [w565]
        tunnel: w525 -> [w563]
        tunnel: w524 -> [w562]
        tunnel: w523 -> [w561]
        stop <- w552 stop-if-true
        n195 = local read "Sample per Channel AI"() -> (w557:dbl)
        n196 = local read "Pulser Cycles"() -> (w564:i32)
        n197 = call-poly <vilib>:"DAQmx Read.vi"("task/channels in"=w559, "number of samples per channel"=w557, "timeout"=-1.0, "error in"=w558) -> ("task out"=w575:refnum<k21>, "data"=w556:dbl[][], "error out"=w574:errorcluster)  [unwired: 9 in]
        n198 = Quotient & Remainder(x=w565, y=w564) -> (x-y*floor(x/y)=w573:i32)  [unwired: 1 out]
        n199 = Equal To 0?(x=w573) -> (x = 0?=w560:bool)
        n200 = Add(x=w556, y=w572) -> (x+y=w569:dbl[][])
        n201 = case shown="True" w560 {
          tunnel: w564 -> [_ w591]
          tunnel: w556 -> [_ _]
          tunnel: w569 -> [w578 w593]
          tunnel: [w578 w592] -> w571
          tunnel: w570 -> [_ w592]
          tunnel: w568 -> [_ w585]
          tunnel: [w576 1 ("Average")] -> w566
          tunnel: w565 -> [w577 _]
          tunnel: w563 -> [_ w587]
          tunnel: w562 -> [_ w589]
          tunnel: w561 -> [_ w588]
          tunnel: [_ w579] -> w553
          frame False {
            n202 = Increment(x=w577) -> (x+1=w576:i32)
          }
          frame True {
            n203 = Divide(x=w593, y=w591) -> (x/y=w580:dbl[][])
            "Hall sensors signal" <- w580
            n204 = for {
              tunnel: w580 -> [w600] mode=indexing
              tunnel: w589 -> [w599]
              tunnel: w588 -> [w598]
              tunnel: w587 -> [w597]
              tunnel: "Offset" -> [w596]
              tunnel: w585 -> [w595]
              tunnel: [w594] -> w584 mode=indexing
              n205 = call "PECT_Feature extraction.vi"("Length T/2"=w595, "Offset"=w596, "Length"=w597, "Start 2"=w598, "Start 1"=w599, "Pulse signal in"=w600) -> ("Feature extraction out"=w594:dbl)  [unwired: 5 in]
            }
            n206 = call "CSV Save.vi"("Array"=w580, "Save Button"="Save Scan mode 2") -> ("Save Status"=w579:bool)  [unwired: 9 in]
            n207 = Index Array(array=w584, index="Sensor No.") -> (element=→"Feature Extraction":dbl)
          }
        }
        n208 = local read "Stop Scan"() -> (w554:bool)
        n209 = Unbundle By Name(w574) -> ("status"=w555:bool)
        n210 = Compound Arithmetic op=OR(w555, w554, w553) -> (w552:bool)
      }
      n211 = while {
        tunnel: w512 -> [w551]
        tunnel: w511 -> [w550]
        tunnel: [w548] -> w509
        tunnel: [w547] -> w510
        stop <- w545 stop-if-true
        n212 = Wait Until Next ms Multiple(millisecond multiple=u32 10) -> ()  [unwired: 1 out]
        n213 = call <vilib>:"DAQmx Is Task Done.vi"("task/channels in"=w551, "error in"=w550) -> ("task out"=w547:refnum<k21>, "error out"=w548:errorcluster)  [unwired: 12 out]
        n214 = local read "Completed"() -> (w544:bool)
        n215 = local read "Stop Scan"() -> (w543:bool)
        n216 = Unbundle By Name(w548) -> ("status"=w546:bool)
        n217 = Compound Arithmetic op=OR(w546, w544, w543) -> (w545:bool)
      }
    }
  }
  n218 = call-poly <vilib>:"DAQmx Create Virtual Channel.vi"("lines"="Digital Line") -> ("task out"=w6:refnum<k21>, "error out"=w7:errorcluster)  [unwired: 13 in]
  n219 = disable-structure shown="Disabled" {
    disable-tunnel: [w607 w608] -> w13
    disable-tunnel: [w606 w609] -> w12
    disable-tunnel: w7 -> [w605 w608]
    disable-tunnel: w6 -> [w604 w609]
    frame Disabled {
      w602 = 10123 items=["Finite Samples"=10178, "Continuous Samples"=10123, "Hardware Timed Single Point"=12522]  # Sample Mode
      n220 = call-poly <vilib>:"DAQmx Timing.vi"("task/channels in"=w604, "sample mode"=w602, "rate"="Digital Sampling Rate", "source"=tag "OnboardClock", "error in"=w605) -> ("task out"=w606:refnum<k21>, "error out"=w607:errorcluster)  [unwired: 9 in]
    }
    frame Enabled {
    }
  }
  n221 = while {
    shift-right: [w625] -> _
    shift-left: T3."No Scan" -> [w626]
    shift-right: [w621] -> _
    shift-left: 0.0 ("Current  Position (mm)") -> [w620]
    shift-right: [w619] -> _
    shift-left: 0.0 ("Current  Position (mm)") -> [w618]
    shift-right: [w617] -> _
    shift-left: 0.0 ("Current  Position (mm)") -> [w616]
    shift-right: [w615] -> _
    shift-left: 0.0 ("Current  Position (mm)") -> [w614]
    shift-right: [w622] -> w60
    shift-left: w117 -> [w624]
    shift-right: [w612] -> w61
    shift-left: w118 -> [w623]
    tunnel: w4 -> [_]
    stop <- w610 stop-if-true
    n222 = case shown="\"Wait to destinatioin Y\"" w626 {
      selector: w626 -> [w637 _ _ _ _]
      tunnel: [w638 T3."Wait to destination X" w702 w719 w775] -> w625
      tunnel: w624 -> [w632 w671 w696 w724 w766]
      tunnel: w623 -> [w631 w670 w695 w723 w765]
      tunnel: [w634 w673 w701 w721 w772] -> w622
      tunnel: [w633 w672 w700 w720 w771] -> w612
      tunnel: [w630 w678 w699 w738 w778] -> w621
      tunnel: w620 -> [w628 w678 w687 w738 w778]
      tunnel: [w636 w677 w704 w737 w777] -> w619
      tunnel: w618 -> [w627 w677 w704 w737 w777]
      tunnel: [w629 w676 w697 w722 w774] -> w617
      tunnel: w616 -> [_ w676 w697 w722 w760]
      tunnel: [w635 w675 w705 w736 w773] -> w615
      tunnel: w614 -> [_ w675 w705 w736 w773]
      frame "No Scan", Default {
        n223 = local read "Scan"() -> (w639:bool)
        n224 = case shown="True" w639 {
          tunnel: [w645 T3."Move X"] -> w638
          tunnel: w637 -> [w645 _]
          tunnel: w632 -> [w644 w651]
          tunnel: w631 -> [w643 w650]
          tunnel: [w644 w656] -> w634
          tunnel: [w643 w655] -> w633
          tunnel: [w642 w647] -> w630
          tunnel: [w641 w646] -> w629
          tunnel: w628 -> [w642 _]
          tunnel: w627 -> [w641 _]
          frame False {
            n225 = Wait (ms)(milliseconds to wait=u32 100) -> ()  [unwired: 1 out]
          }
          frame True {
            n226 = local read "Cur. Pos X"() -> (w653:dbl)
            n227 = local read "Cur. Pos Y"() -> (w654:dbl)
            n228 = local read "Travel per Pulse (mm)"() -> (w652:dbl)
            n229 = call "Sigma_GetPos.vi"("VISA resource name"=w651, "Travel per Pulse (mm)"=w652, "Init Pos X (mm)"=w653, "Init  Pos Y (mm)"=w654, "error in (no error)"=w650) -> ("Pos X (mm)"=w647:dbl, "Pos Y (mm)"=w646:dbl, "VISA resource name out"=w649:refnum<visa-resource-name>, "error out"=w648:errorcluster)  [unwired: 6 in, 1 out]
            "Start Pos. X" <- w647
            "Start. Pos.Y" <- w646
            n230 = local write "Cur. Pos X"(w647) -> ()
            n231 = local write "Cur. Pos Y"(w646) -> ()
            n232 = local read "Travel per Pulse (mm)"() -> (w659:dbl)
            n233 = local read "Step X"() -> (w660:dbl)
            n234 = local write "Direction (+)"(TRUE ("Direction (+)")) -> ()
            n235 = local write "Move X"(TRUE ("Move X")) -> ()
            n236 = call "Sigma_TriggerOut.vi"("Axis(1)"=1, "error in (no error)"=w648, "Trigger distance (mm)"=w660, "Travel per Pulse (mm)"=w659, "VISA resource name"=w649) -> ("error out"=w657:errorcluster, "VISA resource name out"=w658:refnum<visa-resource-name>)  [unwired: 5 in]
            n237 = flat-sequence {
              tunnel: [w667] -> w656
              tunnel: w658 -> [w667]
              tunnel: [w666] -> w655
              tunnel: w657 -> [w666]
              frame #0 {
                n238 = Wait (ms)(milliseconds to wait=u32 100) -> ()  [unwired: 1 out]
              }
            }
          }
        }
        n239 = local read "X-length"() -> (w636:dbl)
        n240 = local read "Step Y"() -> (w635:dbl)
      }
      frame "Move X" {
        n241 = local read "Travel per Pulse (mm)"() -> (w680:dbl)
        n242 = local read "X-length"() -> (w681:dbl)
        n243 = call "Sigma_MoveAbs.vi"("Direction (+)"="Direction (+)", "Axis (1)"=1, "error in (no error)"=w670, "Travel (1mm)"=w681, "Travel per Pulse (0.004mm)"=w680, "VISA resource name"=w671) -> ("error out"=w668:errorcluster, "VISA resource name out"=w669:refnum<visa-resource-name>)  [unwired: 4 in]
        n244 = flat-sequence {
          tunnel: [w685] -> w673
          tunnel: w669 -> [w685]
          tunnel: [w684] -> w672
          tunnel: w668 -> [w684]
          frame #0 {
            n245 = Wait (ms)(milliseconds to wait=u32 100) -> ()  [unwired: 1 out]
          }
        }
      }
      frame "Wait to destination X" {
        n246 = local read "Cur. Pos X"() -> (w692:dbl)
        n247 = local read "Cur. Pos Y"() -> (w691:dbl)
        n248 = local read "Travel per Pulse (mm)"() -> (w698:dbl)
        n249 = call "Sigma_GetPos.vi"("VISA resource name"=w696, "Travel per Pulse (mm)"=w698, "Init Pos X (mm)"=w692, "Init  Pos Y (mm)"=w691, "error in (no error)"=w695) -> ("Pos X (mm)"=w686:dbl, "Pos Y (mm)"=w690:dbl, "VISA resource name out"=w694:refnum<visa-resource-name>, "error out"=w693:errorcluster)  [unwired: 6 in, 1 out]
        n250 = Absolute Value(x=w704) -> (abs(x)=w706:dbl)
        n251 = local write "Cur. Pos X"(w686) -> ()
        n252 = local write "Cur. Pos Y"(w690) -> ()
        n253 = Subtract(x=w686, y=w687) -> (x-y=w708:dbl)
        n254 = Absolute Value(x=w708) -> (abs(x)=w707:dbl)
        n255 = Subtract(x=w707, y=w706) -> (x-y=w689:dbl)
        n256 = call "Convert Double Precision.vi"("Input"=w689) -> ("Output"=w688:dbl)  [unwired: 10 in]
        n257 = Greater Or Equal To 0?(x=w688) -> (x >= 0?=w703:bool)
        n258 = case shown="True" w703 {
          tunnel: [T3."Wait to destination X" T3."Move Y"] -> w702
          tunnel: w694 -> [w711 w715]
          tunnel: w693 -> [w710 w714]
          tunnel: [w711 w715] -> w701
          tunnel: [w710 w714] -> w700
          tunnel: [w709 w716] -> w699
          tunnel: w687 -> [w709 _]
          frame False {
            n259 = disable-structure shown="비활성화" {
              frame Disabled {
                n260 = Wait (ms)(milliseconds to wait=u32 100) -> ()  [unwired: 1 out]
              }
              frame Enabled {
              }
            }
          }
          frame True {
            n261 = local read "Cur. Pos X"() -> (w716:dbl)
            n262 = local write "Move X"(FALSE ("Move X")) -> ()
          }
        }
      }
      frame "Move Y" {
        n263 = local read "Y-length"() -> (w727:dbl)
        n264 = local read "Step Y"() -> (w725:dbl)
        n265 = local read "Start. Pos.Y"() -> (w730:dbl)
        n266 = Subtract(x=w727, y=w725) -> (x-y=w726:dbl)
        n267 = Subtract(x=w730, y=w722) -> (x-y=w735:dbl)
        n268 = Absolute Value(x=w726) -> (abs(x)=w733:dbl)
        n269 = Absolute Value(x=w735) -> (abs(x)=w734:dbl)
        n270 = Subtract(x=w734, y=w733) -> (x-y=w728:dbl)
        n271 = local write "Move X"(FALSE ("Move X")) -> ()
        n272 = call "Convert Double Precision.vi"("Input"=w728) -> ("Output"=w729:dbl)  [unwired: 10 in]
        n273 = Greater Or Equal To 0?(x=w729) -> (x >= 0?=w731:bool)
        n274 = case shown="False" w731 {
          tunnel: [w741 w757] -> w721
          tunnel: [w740 w756] -> w720
          tunnel: w724 -> [w743 w755]
          tunnel: w723 -> [w742 w754]
          tunnel: [T3."Wait to destinatioin Y" T3."No Scan"] -> w719
          frame False {
            n275 = local read "Travel per Pulse (mm)"() -> (w747:dbl)
            n276 = local read "Step Y"() -> (w748:dbl)
            n277 = call "Sigma_MoveAbs.vi"("Direction (+)"=TRUE, "Axis (1)"=2, "error in (no error)"=w742, "Travel (1mm)"=w748, "Travel per Pulse (0.004mm)"=w747, "VISA resource name"=w743) -> ("error out"=w745:errorcluster, "VISA resource name out"=w746:refnum<visa-resource-name>)  [unwired: 4 in]
            n278 = flat-sequence {
              tunnel: [w752] -> w741
              tunnel: w746 -> [w752]
              tunnel: [w751] -> w740
              tunnel: w745 -> [w751]
              frame #0 {
                n279 = Wait (ms)(milliseconds to wait=u32 100) -> ()  [unwired: 1 out]
              }
            }
          }
          frame True {
            n280 = call "Sigma_TriggerOff.vi"("error in (no error)"=w754, "VISA resource name"=w755) -> ("error out"=w756:errorcluster, "VISA resource name out"=w757:refnum<visa-resource-name>)  [unwired: 8 in]
            n281 = local write "Scan"(FALSE ("Move X")) -> ()
          }
        }
      }
      frame "Wait to destinatioin Y" {
        n282 = local read "Cur. Pos X"() -> (w769:dbl)
        n283 = local read "Cur. Pos Y"() -> (w768:dbl)
        n284 = local read "Travel per Pulse (mm)"() -> (w770:dbl)
        n285 = call "Sigma_GetPos.vi"("VISA resource name"=w766, "Travel per Pulse (mm)"=w770, "Init Pos X (mm)"=w769, "Init  Pos Y (mm)"=w768, "error in (no error)"=w765) -> ("Pos X (mm)"=w767:dbl, "Pos Y (mm)"=w759:dbl, "VISA resource name out"=w764:refnum<visa-resource-name>, "error out"=w763:errorcluster)  [unwired: 6 in, 1 out]
        n286 = Absolute Value(x=w773) -> (abs(x)=w779:dbl)
        n287 = Subtract(x=w759, y=w760) -> (x-y=w781:dbl)
        n288 = local write "Cur. Pos X"(w767) -> ()
        n289 = local write "Cur. Pos Y"(w759) -> ()
        n290 = Absolute Value(x=w781) -> (abs(x)=w780:dbl)
        n291 = Subtract(x=w780, y=w779) -> (x-y=w762:dbl)
        n292 = call "Convert Double Precision.vi"("Input"=w762) -> ("Output"=w761:dbl)  [unwired: 10 in]
        n293 = Greater Or Equal To 0?(x=w761) -> (x >= 0?=w776:bool)
        n294 = case shown="False" w776 {
          tunnel: [T3."Wait to destinatioin Y" T3."Move X"] -> w775
          tunnel: w760 -> [w784 _]
          tunnel: [w784 w791] -> w774
          tunnel: [w783 w790] -> w772
          tunnel: [w782 w789] -> w771
          tunnel: w764 -> [w783 w790]
          tunnel: w763 -> [w782 w789]
          frame False {
            n295 = disable-structure shown="비활성화" {
              frame Disabled {
                n296 = Wait (ms)(milliseconds to wait=u32 100) -> ()  [unwired: 1 out]
              }
              frame Enabled {
              }
            }
          }
          frame True {
            n297 = local read "Cur. Pos Y"() -> (w791:dbl)
            n298 = local read "Direction (+)"() -> (w788:bool)
            n299 = local write "Move X"(TRUE ("Move X")) -> ()
            n300 = Not(x=w788) -> (.not. x?=w787:bool)
            n301 = local write "Direction (+)"(w787) -> ()
          }
        }
      }
    }
    n302 = Unbundle By Name(w612) -> ("status"=w611:bool)
    n303 = local read "Stop Scan"() -> (w613:bool)
    n304 = Compound Arithmetic op=OR(w611, w613) -> (w610:bool)
  }
  n305 = while {
    shift-right: [w796] -> _
    shift-left: w117 -> [w801]
    shift-right: [w798] -> _
    shift-left: w118 -> [w800]
    stop <- w797 stop-if-true
    n306 = event shown="[0] Timeout" {
      selector: _ -> [_ _ _ _ _ _ _ _ _ _ _]
      dyn-events: _ -> [_ _ _ _ _ _ _ _ _ _ _]
      timeout: 100 -> [_ _ _ _ _ _ _ _ _ _ _]
      tunnel: w801 -> [w806 w839 w852 w855 w870 w885 w900 w917 w929 w939 w951]
      tunnel: w800 -> [w805 w838 w849 w854 w869 w884 w899 w916 w928 w938 w950]
      tunnel: [w804 w839 w851 w857 w872 w887 w902 w914 w927 w941 w953] -> w796
      tunnel: [w803 w838 w850 w856 w871 w886 w901 w913 w926 w940 w952] -> w798
      tunnel: [_ "Stop Scan" _ _ _ _ _ _ _ _ _] -> w795
      event Timeout {
        n307 = event-data() -> ()  [unwired: 1 in, 2 out]
        n308 = local read "Scan"() -> (w802:bool)
        n309 = case shown="False" w802 {
          tunnel: w806 -> [w818 w837]
          tunnel: w805 -> [w817 w836]
          tunnel: [w816 w837] -> w804
          tunnel: [w815 w836] -> w803
          frame False {
            # "Stop at LS"
            n310 = local read "Travel per Pulse (mm)"() -> (w810:dbl)
            n311 = local read "Cur. Pos X"() -> (w808:dbl)
            n312 = local read "Cur. Pos Y"() -> (w807:dbl)
            n313 = call "Sigma_GetPos.vi"("VISA resource name"=w818, "Travel per Pulse (mm)"=w810, "Init Pos X (mm)"=w808, "Init  Pos Y (mm)"=w807, "error in (no error)"=w817) -> ("Pos X (mm)"=w813:dbl, "Pos Y (mm)"=w814:dbl, "VISA resource name out"=w811:refnum<visa-resource-name>, "State String"=w809:string, "error out"=w812:errorcluster)  [unwired: 6 in]
            n314 = local write "Cur. Pos X"(w813) -> ()
            n315 = local write "Cur. Pos Y"(w814) -> ()
            n316 = case shown="\"W\"" w809 {
              tunnel: [w820 w825 w830 w835] -> w816
              tunnel: [w819 w824 w829 w834] -> w815
              tunnel: w811 -> [w820 w822 w827 w832]
              tunnel: w812 -> [w819 w821 w826 w831]
              frame "K", Default {
              }
              frame "L" {
                n317 = call "Sigma_Stop.vi"("Axis (1)"="1", "error in (no error)"=w821, "VISA resource name"=w822) -> ("error out"=w824:errorcluster, "VISA resource name out"=w825:refnum<visa-resource-name>)  [unwired: 7 in]
              }
              frame "M" {
                n318 = call "Sigma_Stop.vi"("Axis (1)"="2", "error in (no error)"=w826, "VISA resource name"=w827) -> ("error out"=w829:errorcluster, "VISA resource name out"=w830:refnum<visa-resource-name>)  [unwired: 7 in]
              }
              frame "W" {
                n319 = call "Sigma_Stop.vi"("Axis (1)"="W", "error in (no error)"=w831, "VISA resource name"=w832) -> ("error out"=w834:errorcluster, "VISA resource name out"=w835:refnum<visa-resource-name>)  [unwired: 7 in]
              }
            }
          }
          frame True {
          }
        }
      }
      event "Stop Scan": Value Change {
        n320 = event-data() -> ()  [unwired: 1 in, 2 out]
      }
      event "Save Speed": Value Change {
        n321 = event-data() -> ()  [unwired: 1 in, 5 out]
        n322 = local read "Travel per Pulse (mm)"() -> (w841:dbl)
        n323 = local read "1  Max"() -> (w846:dbl)
        n324 = local read "1 Rate"() -> (w845:dbl)
        n325 = local read "2 Rate"() -> (w842:dbl)
        n326 = local read "2 Max"() -> (w843:dbl)
        n327 = local read "1 Min"() -> (w847:dbl)
        n328 = local read "2 Min"() -> (w844:dbl)
        n329 = call "Sigma_SetSpeed.vi"("VISA resource name"=w852, "Travel per Pulse (0.004mm)"=w841, "Min (1mm) 2"=w844, "Max (2mm) 2"=w843, "Rate (1mm) 2"=w842, "error in (no error)"=w849, "Axis (1)"="W", "Min (1mm)"=w847, "Max (2mm)"=w846, "Rate (1mm)"=w845) -> ("VISA resource name out"=w851:refnum<visa-resource-name>, "error out"=w850:errorcluster)  [unwired: 8 in]
      }
      event "Right": Value Change {
        n330 = event-data() -> ()  [unwired: 1 in, 1 out]
        n331 = case shown="True" "Right" {
          tunnel: [w859 w865] -> w857
          tunnel: [w858 w864] -> w856
          tunnel: w855 -> [w859 w867]
          tunnel: w854 -> [w858 w866]
          frame False {
          }
          frame True {
            n332 = local read "Travel per Pulse (mm)"() -> (w861:dbl)
            n333 = local read "Move Distance"() -> (w860:dbl)
            n334 = call "Sigma_MoveAbs.vi"("Direction (+)"=FALSE, "Axis (1)"=1, "error in (no error)"=w866, "Travel (1mm)"=w860, "Travel per Pulse (0.004mm)"=w861, "VISA resource name"=w867) -> ("error out"=w864:errorcluster, "VISA resource name out"=w865:refnum<visa-resource-name>)  [unwired: 4 in]
          }
        }
      }
      event "Left": Value Change {
        n335 = event-data() -> ()  [unwired: 1 in, 1 out]
        n336 = case shown="True" "Left" {
          tunnel: [w874 w881] -> w872
          tunnel: [w873 w880] -> w871
          tunnel: w870 -> [w874 w882]
          tunnel: w869 -> [w873 w879]
          frame False {
          }
          frame True {
            n337 = local read "Travel per Pulse (mm)"() -> (w876:dbl)
            n338 = local read "Move Distance"() -> (w875:dbl)
            n339 = call "Sigma_MoveAbs.vi"("Direction (+)"=TRUE, "Axis (1)"=1, "error in (no error)"=w879, "Travel (1mm)"=w875, "Travel per Pulse (0.004mm)"=w876, "VISA resource name"=w882) -> ("error out"=w880:errorcluster, "VISA resource name out"=w881:refnum<visa-resource-name>)  [unwired: 4 in]
          }
        }
      }
      event "Front": Value Change {
        n340 = event-data() -> ()  [unwired: 1 in, 1 out]
        n341 = case shown="True" "Front" {
          tunnel: [w889 w895] -> w887
          tunnel: [w888 w894] -> w886
          tunnel: w885 -> [w889 w897]
          tunnel: w884 -> [w888 w896]
          frame False {
          }
          frame True {
            n342 = local read "Travel per Pulse (mm)"() -> (w891:dbl)
            n343 = local read "Move Distance"() -> (w890:dbl)
            n344 = call "Sigma_MoveAbs.vi"("Direction (+)"=FALSE, "Axis (1)"=2, "error in (no error)"=w896, "Travel (1mm)"=w890, "Travel per Pulse (0.004mm)"=w891, "VISA resource name"=w897) -> ("error out"=w894:errorcluster, "VISA resource name out"=w895:refnum<visa-resource-name>)  [unwired: 4 in]
          }
        }
      }
      event "Back": Value Change {
        n345 = event-data() -> ()  [unwired: 1 in, 1 out]
        n346 = case shown="True" "Back" {
          tunnel: [w904 w910] -> w902
          tunnel: [w903 w909] -> w901
          tunnel: w900 -> [w904 w912]
          tunnel: w899 -> [w903 w911]
          frame False {
          }
          frame True {
            n347 = local read "Travel per Pulse (mm)"() -> (w906:dbl)
            n348 = local read "Move Distance"() -> (w905:dbl)
            n349 = call "Sigma_MoveAbs.vi"("Direction (+)"=TRUE, "Axis (1)"=2, "error in (no error)"=w911, "Travel (1mm)"=w905, "Travel per Pulse (0.004mm)"=w906, "VISA resource name"=w912) -> ("error out"=w909:errorcluster, "VISA resource name out"=w910:refnum<visa-resource-name>)  [unwired: 4 in]
          }
        }
      }
      event "Home X": Value Change {
        n350 = event-data() -> ()  [unwired: 1 in, 1 out]
        n351 = case shown="True" "Home X" {
          tunnel: [w919 w922] -> w914
          tunnel: [w918 w921] -> w913
          tunnel: w917 -> [w919 w924]
          tunnel: w916 -> [w918 w923]
          frame False {
          }
          frame True {
            n352 = call "Sigma_Home.vi"("Axis (1)"="1", "error in (no error)"=w923, "VISA resource name"=w924) -> ("error out"=w921:errorcluster, "VISA resource name out"=w922:refnum<visa-resource-name>)  [unwired: 7 in]
          }
        }
      }
      event "Home Y": Value Change {
        n353 = event-data() -> ()  [unwired: 1 in, 1 out]
        n354 = case shown="True" "Home Y" {
          tunnel: [w931 w934] -> w927
          tunnel: [w930 w933] -> w926
          tunnel: w929 -> [w931 w936]
          tunnel: w928 -> [w930 w935]
          frame False {
          }
          frame True {
            n355 = call "Sigma_Home.vi"("Axis (1)"="2", "error in (no error)"=w935, "VISA resource name"=w936) -> ("error out"=w933:errorcluster, "VISA resource name out"=w934:refnum<visa-resource-name>)  [unwired: 7 in]
          }
        }
      }
      event "Stop 3": Value Change {
        n356 = event-data() -> ()  [unwired: 1 in, 1 out]
        n357 = case shown="True" "Stop 3" {
          tunnel: [w943 w944] -> w941
          tunnel: [w942 w945] -> w940
          tunnel: w939 -> [w943 w947]
          tunnel: w938 -> [w942 w946]
          frame False {
          }
          frame True {
            n358 = call "Sigma_Stop.vi"("Axis (1)"="W", "error in (no error)"=w946, "VISA resource name"=w947) -> ("error out"=w945:errorcluster, "VISA resource name out"=w944:refnum<visa-resource-name>)  [unwired: 7 in]
          }
        }
      }
      event "Emergency Stop": Value Change {
        n359 = event-data() -> ()  [unwired: 1 in, 1 out]
        n360 = case shown="True" "Emergency Stop" {
          tunnel: [w955 w958] -> w953
          tunnel: [w954 w957] -> w952
          tunnel: w951 -> [w955 w960]
          tunnel: w950 -> [w954 w959]
          frame False {
          }
          frame True {
            n361 = call "Sigma_Stop.vi"("Axis (1)"="E", "error in (no error)"=w959, "VISA resource name"=w960) -> ("error out"=w957:errorcluster, "VISA resource name out"=w958:refnum<visa-resource-name>)  [unwired: 7 in]
          }
        }
      }
    }
    n362 = Unbundle By Name(w798) -> ("status"=w799:bool)
    n363 = Compound Arithmetic op=OR(w799, w795) -> (w797:bool)
  }
  n364 = local read "Counter Status"() -> (w10:bool)
  n365 = call <vilib>:"DAQmx Start Task.vi"("task/channels in"=w12, "error in"=w13) -> ("task out"=w9:refnum<k21>, "error out"=w8:errorcluster)  [unwired: 12 in]
  n366 = while {
    tunnel: [w974] -> w2
    tunnel: [w962] -> w1
    tunnel: w8 -> [w973]
    tunnel: w9 -> [w972]
    shift-right: [w967] -> _
    shift-left: w10 -> [w971]
    shift-right: [w961] -> _
    shift-left: 0.0 -> [w970]
    tunnel: w4 -> [_]
    stop <- w963 stop-if-true
    # "Rising edge"
    n367 = call-poly <vilib>:"DAQmx Read.vi"("task/channels in"=w972, "error in"=w973) -> ("task out"=w974:refnum<k21>, "data"=w967:bool, "error out"=w962:errorcluster)  [unwired: 11 in]
    "Counter Status" <- w967
    n368 = Not Equal?(x=w971, y=w967) -> (x != y?=w969:bool)
    n369 = And(x=w969, y=w967) -> (x .and. y?=w968:bool)
    n370 = case shown="True" w968 {
      tunnel: w970 -> [w975 w977]
      tunnel: [w975 w976] -> w961
      frame False {
      }
      frame True {
        n371 = Increment(x=w977) -> (x+1=w976:dbl)
      }
    }
    n372 = local write "Motor Pulse Count"(w961) -> ()
    n373 = local read "Completed"() -> (w965:bool)
    n374 = local read "Stop Scan"() -> (w966:bool)
    n375 = Unbundle By Name(w962) -> ("status"=w964:bool)
    n376 = Compound Arithmetic op=OR(w964, w965, w966) -> (w963:bool)
  }
  n377 = call <vilib>:"DAQmx Clear Task.vi"("task in"=w2, "error in"=w1) -> ("error out"=w3:errorcluster)  [unwired: 13 in]
  n378 = call <vilib>:"Simple Error Handler.vi"("error in (no error)"=w3) -> ()  [unwired: 4 in, 5 out]
  n379 = VISA Close(VISA resource name=w60, error in (no error)=w61) -> (error out=w59:errorcluster)
  n380 = call <vilib>:"Simple Error Handler.vi"("error in (no error)"=w59) -> ()  [unwired: 4 in, 5 out]
  n381 = call <vilib>:"DAQmx Clear Task.vi"("task in"=w83, "error in"=w82) -> ("error out"=w89:errorcluster)  [unwired: 13 in]
  n382 = call <vilib>:"Simple Error Handler.vi"("error in (no error)"=w89) -> ()  [unwired: 4 in, 5 out]
  n383 = call <vilib>:"DAQmx Clear Task.vi"("task in"=w21, "error in"=w20) -> ("error out"=w22:errorcluster)  [unwired: 13 in]
  n384 = call <vilib>:"Simple Error Handler.vi"("error in (no error)"=w22) -> ()  [unwired: 4 in, 5 out]
  n385 = call <vilib>:"Simple Error Handler.vi"() -> ()  [unwired: 5 in, 5 out]
  "Move X" <- FALSE ("Move X")
